vi "main.vi"() -> ()   [LabVIEW 2014]
uses:
  <vilib>/Utility/error.llb/DialogType.ctl
panel:
  in  "stop 2":bool
  out "Waveform Chart 2":cluster{"number: 0 to 1":dbl, dbl}(graph)
  out "Ostatnia wartość":dbl
  out "Średnia":dbl
  out "Pomiary":dbl[](array[numeric])
  out "Waveform Chart":dbl(graph)
  in  "stop":bool
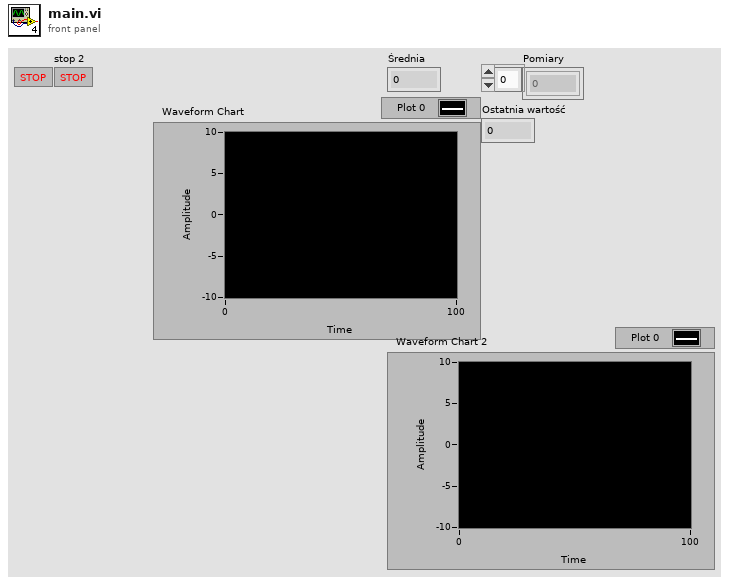
[diagram p1: front panel]
types:
  T1 = typedef "DialogType.ctl" = u16
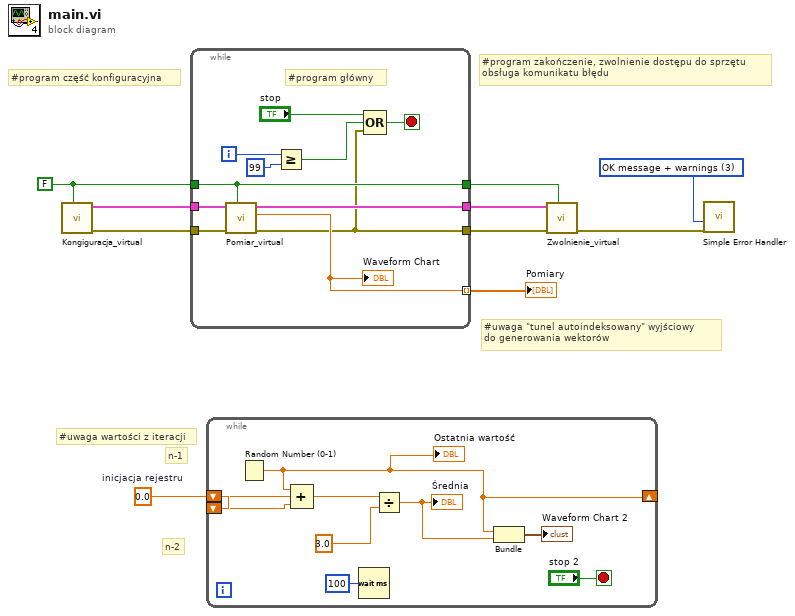
[diagram p0: block diagram]
diagram:
  w1 = 0.0  # inicjacja rejestru
  w3 = T1 3 items=["no dialog", "OK message", "continue or stop message", "OK message + warnings", "continue/stop + warnings"] ("type of dialog (OK msg:1)")
  w8 = FALSE ("Error Generate")
  # "n-2"
  # "n-1"
  # "#uwaga wartości z iteracji"
  # "#uwaga \"tunel autoindeksowany\" wyjściowy\ndo generowania wektorów"
  # "#program zakończenie, zwolnienie dostępu do sprzętu\nobsługa komunikatu błędu"
  # "#program część konfiguracyjna"
  n1 = call "Kongiguracja_virtual.vi"("Error Generate"=w8) -> ("error out"=w10:errorcluster, "Reference out"=w9:cluster{"Numeric":dbl, "Boolean":bool})  [unwired: 9 in]
  n2 = while {
    tunnel: w10 -> [w21]
    tunnel: w9 -> [w20]
    tunnel: w8 -> [w18]
    tunnel: [w19] -> w7
    tunnel: [w11] -> w6
    tunnel: [w18] -> w5
    tunnel: [w13] -> w2 mode=indexing
    i -> [w15]
    stop <- w16 stop-if-true
    # "#program główny"
    n3 = call "Pomiar_virtual.vi"("Error Generate"=w18, "error in (no error)"=w21, "Reference in"=w20) -> ("error out"=w11:errorcluster, "out"=w13:dbl, "Reference out"=w19:cluster{"Numeric":dbl, "Boolean":bool})  [unwired: 6 in]
    "Waveform Chart" <- w13
    n4 = Greater Or Equal?(x=w15, y=99) -> (x >= y?=w12:bool)
    n5 = Compound Arithmetic op=OR("stop", w12, w11) -> (w16:bool)
  }
  "Pomiary" <- w2
  n6 = while {
    shift-right: [w26] -> _
    shift-left: w1 -> [w30]
    shift-left: w1 -> [w29]
    stop <- "stop 2" stop-if-true
    n7 = Random Number (0-1)() -> (number: 0 to 1=w26:dbl)
    "Ostatnia wartość" <- w26
    n8 = Compound Arithmetic op=ADD(w26, w30, w29) -> (w28:dbl)
    n9 = Wait (ms)(milliseconds to wait=u32 100) -> ()  [unwired: 1 out]
    n10 = Divide(x=w28, y=3.0) -> (x/y=w25:dbl)
    "Średnia" <- w25
    n11 = Bundle "Bundle"("number: 0 to 1"=w26, w25) -> (→"Waveform Chart 2":cluster{"number: 0 to 1":dbl, dbl})  [unwired: 1 in]
  }
  n12 = call "Zwolnienie_virtual.vi"("Error Generate"=w5, "error in (no error)"=w6, "Reference in"=w7) -> ("error out"=w4:errorcluster)  [unwired: 8 in]
  n13 = call <vilib>:"Simple Error Handler.vi"("type of dialog (OK msg:1)"=w3, "error in (no error)"=w4) -> ()  [unwired: 3 in, 5 out]
